vi "Actor Core.vi"(8 "error in":errorcluster, 11 "Project Builder in":refnum<class "Project Builder.lvclass">) -> (0 "error out":errorcluster, 3 "Actor out":refnum<class "Actor.lvclass">)   [LabVIEW 2014, in "Project Builder.lvclass"]
doc: "(<B>Filename</B>: Actor Framework.lvlib:Actor.lvclass:Actor Core.vi)\n\nReceives messages to the actor, reacts to them, and initiates any error handling that may shut the actor down.\n\nDescendant classes may override this VI to append parallel tasks for the actor to complete while it handles messages. Overrides use the Call Parent Method node."
uses:
  Project Builder.lvclass
  Controls/Source Code Control Selection - STYP.ctl
  Controls/Cron String - STYP.ctl
  <vilib>/ActorFramework/Actor/Actor.lvclass
  Jenkins Builder/Jenkins Builder.lvclass
  QSM/TypeDef/Invalid Option - STYP.ctl
  Project Builder.lvclass/Project Builder.ctl
  <vilib>/Utility/miscctls.llb/LVRowAndColumnTypeDef.ctl
  Shared/Controls/LabVIEW Build - STYP.ctl
  Shared/Controls/Run VI - STYP.ctl
  Actors/CI Project/CI Project.lvclass
  <vilib>/ActorFramework/Actor/Actor.lvclass/Actor.ctl
  <vilib>/ActorFramework/Message Enqueuer/Message Enqueuer.lvclass/Message Enqueuer.ctl
  Actors/Job Initialize/Job Initialize.lvclass
  Actors/CI Project/CI Project.lvclass/CI Project.ctl
  Actors/Job Initialize/Job Initialize.lvclass/Job Initialize.ctl
  Actors/Build Job/Build Job.lvclass
  Jenkins Builder Messages/Build Msg/Build Msg.lvclass/Build Msg.ctl
  Actors/CI Project/Read Build Recipe.vi
  Actors/CI Project/Read Project Name.vi
  Actors/CI Project/Read Artifact Days.vi
  Actors/CI Project/Read HostName.vi
  Actors/CI Project/Read Notification.vi
  Actors/Job Initialize/Read Build Trigger.vi
  Actors/Job Initialize/Read Source Code Poll.vi
  <vilib>/ActorFramework/Message Enqueuer/Init from Existing Queue.vi
  <vilib>/ActorFramework/Message Enqueuer/Enqueue.vi
  QSM/API/QSM - Add State(s) to Back.vi
  <vilib>/ActorFramework/Message Priority Queue/Priority Enqueue.vi
  QSM/API/QSM - Add State(s) to Front.vi
  <vilib>/ActorFramework/Message Enqueuer/Message Enqueuer.lvclass
  <vilib>/ActorFramework/Stop Msg/Stop Msg.lvclass
  Jenkins Builder Messages/Build Msg/Build Msg.lvclass
  Actors/LabVIEW Build/LabVIEW Build.lvclass
  Actors/Run VI/Run VI.lvclass
panel:
  in  "Load":bool
  in  "Save":bool
  in  "Build":bool
  in  "Main Tab":enum32{"Information", "Result Text"}(tab)
  out "Build Type Tab":enum32{"LabVIEW Build", "Run VI", "Blank"}(tab)
  in  "Title 2":string="LabVIEW Build"
  in  "Project Path":path=path "C:/Projects/LabVIEW Continuous Integration/LabVIEW Continuous Integration.lvproj"
  in  "Build Spec":u16(ring) items=["LabVIEW CI Service", "Test CI Mediator", "Test LabVIEW Launcher"]
  in  "Wait Until Done?":bool
  in  "VI Path":path=path "C:/Projects/LabVIEW Continuous Integration/LabVIEW Continuous Integration.lvproj"
  in  "Title 3":string="Run VI"
  in  "Source Code Poll":T1
  in  "Build Trigger":T2={"Day of Week"=enum."Everyday", "Hour"=23, "Enable?"=FALSE} {"Hour" min=0 max=23}
  in  "Jenkins Hostname(IP Address:Port Number)":string
  in  "Project Name":string="LabVIEW Test"
  in  "How many days to Artifact?":i32=15
  in  "Notification (Separate by Space)":string="brandyn.adderley@ni.com"
  in  "Build Steps":i32(listbox) caption="Build Steps(2)"
  in  "Add":bool
  in  "Remove":bool
  in  "Step Type":enum16{"LabVIEW Build", "Run VI"}(ring)
  out "Build Text":string
  out "Progress":u8(slide) scale=0.0..100.0
  in  "Title":string="Continuous Integration Project"
  # "<No build Steps>"
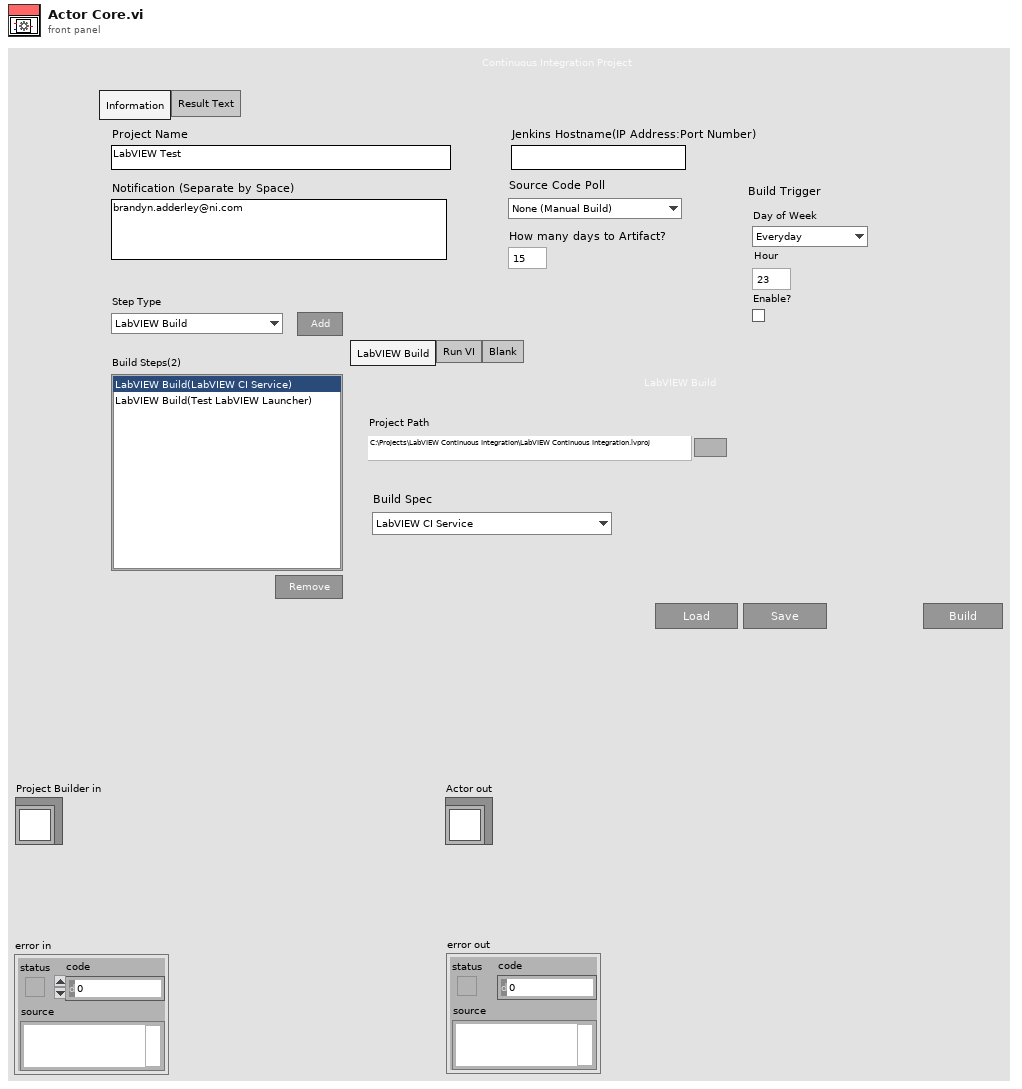
[diagram p1: front panel]
types:
  T1 = typedef "Source Code Control Selection - STYP.ctl" = enum16{"None (Manual Build)", "Every 15 Minutes", "Every 30 Minutes", "Every 45 Minutes", "Every Hour", "Every 2 Hours", "Everyday "}
  T2 = typedef "Cron String - STYP.ctl" = cluster{"Day of Week":enum16{"Everyday", "Sunday", "Monday", "Tuesday", "Wednesday", "Thursday", "Friday", "Saturday"}, "Hour":i32, "Enable?":bool}
  T3 = typedef "Invalid Option - STYP.ctl" = enum16{"Dialog", "Error", "Ignore"}
  T4 = typedef "QSM - STYP.ctl" = cluster{"Invalid Option":T3, "QSM":refnum<queue>}
  T5 = enum8{"Enabled", "Disabled", "Disabled and Grayed Out"}
  T6 = typedef "LVRowAndColumnTypeDef.ctl" = cluster{"Row":i32, "Column":i32}
  T7 = typedef "LabVIEW Build - STYP.ctl" = cluster{"Executor_Number":string, "Workspace_Path":string, "Build_Spec":string, "Project_Path":string, "Auto_Version_Increment":bool}
  T8 = typedef "Run VI - STYP.ctl" = cluster{"Executor_Number":string, "VI_Path":string, "Wait_Until_Done":bool}
  T9 = enum32{"invalid app kind", "Development System", "Run Time System", "Student Edition", "Embedded LabVIEW", "Evaluation", "Custom"}
  T10 = enum16{"open", "replace", "create", "open or create", "replace or create", "replace or create with confirmation"}
  T11 = cluster{"Core":cluster{"Current VI Reference":refnum<vi>, "Close Panel on Exit?":bool}, "Project Name":string, "Jenkins Hostname":string, "Notification":string, "How many days to Artifact?":i32, "Source Code Poll":T1, "Build Trigger":T2, "Main Tab":enum32{"Information", "Result Text"}, "Build Steps Ref":refnum<vi>, "Build Type Tab":enum32{"LabVIEW Build", "Run VI", "Blank"}, "Project Path Ref":refnum<vi>, "Build Spec":refnum<vi>, "Number of Build Steps":i32, "Step Type":enum16{"LabVIEW Build", "Run VI"}, "Active Step Data":variant, "Build Steps Data":variant, "Active GUID":string, "Build Step Index":i32, "Build Events":refnum<event-registration>, "CI Project":refnum<class "CI Project.lvclass">, "Build Text":string, "Jenkins Build Count":i32, "Jenkins Steps":i32, "Build Ref":refnum<vi>, "Load Ref":refnum<vi>, "Save Ref":refnum<vi>, "List Text":string}
  T12 = cluster{"Current VI Reference":refnum<vi>, "Close Panel on Exit?":bool}
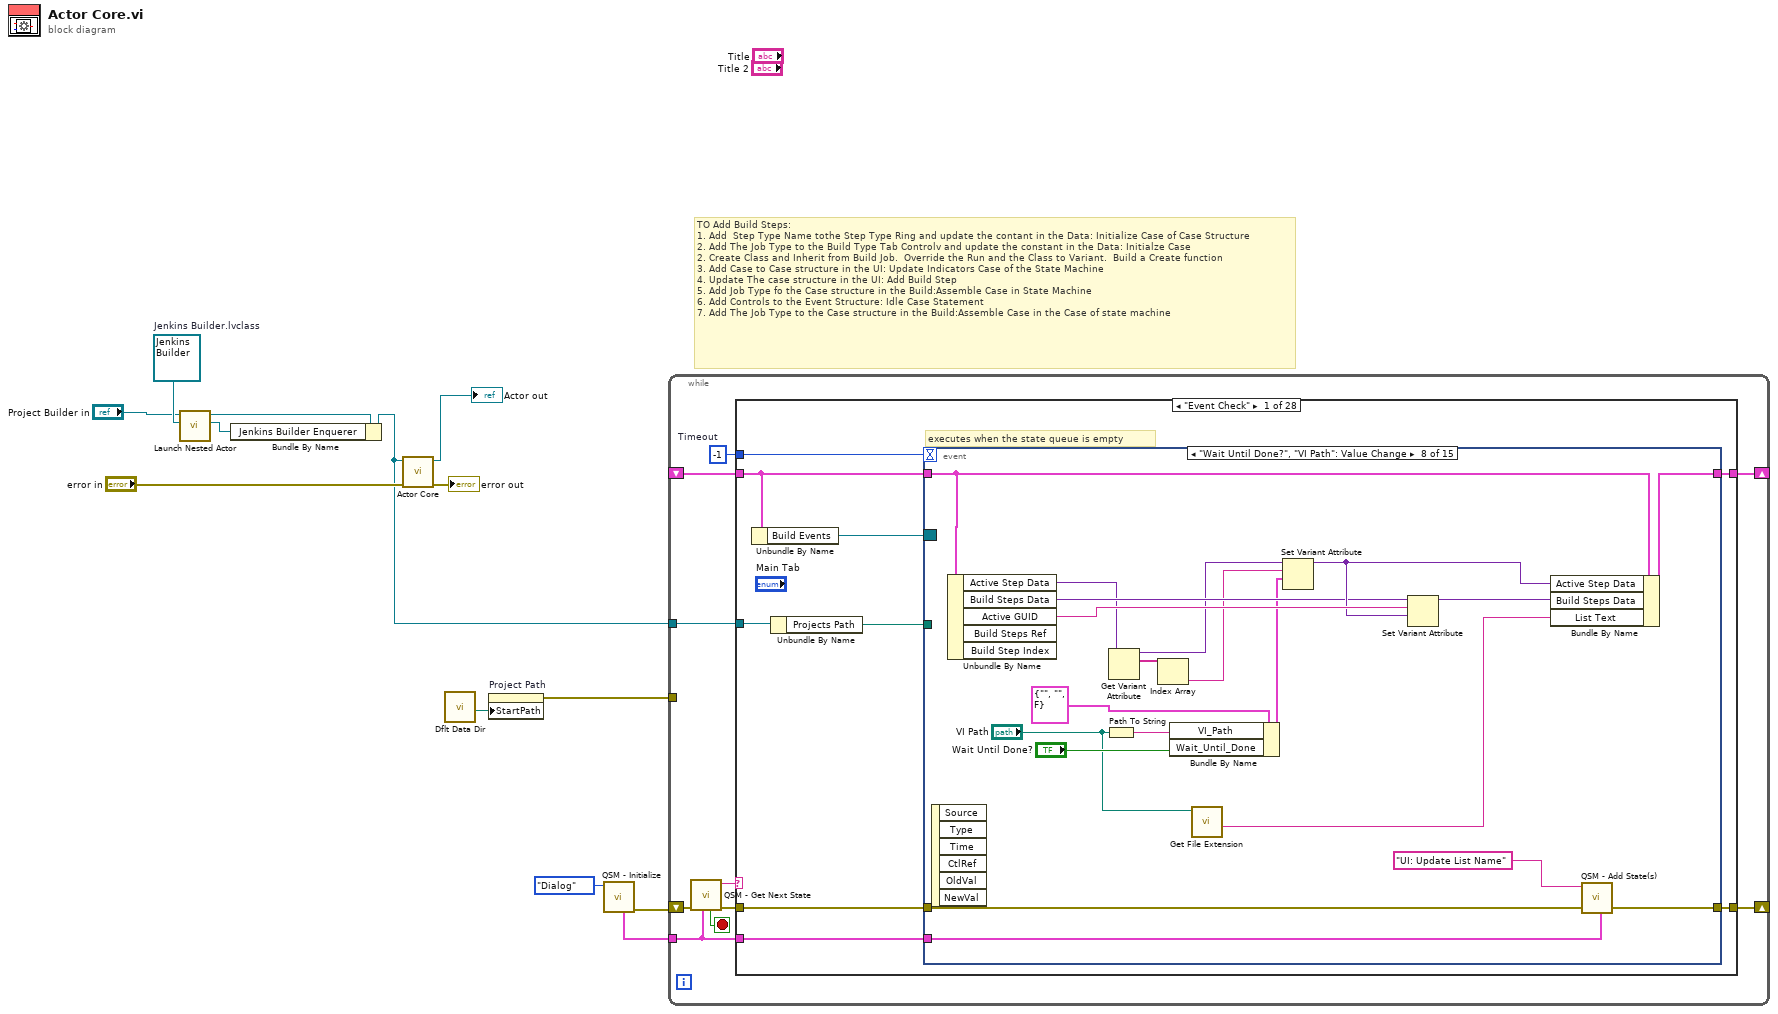
[diagram p0: block diagram]
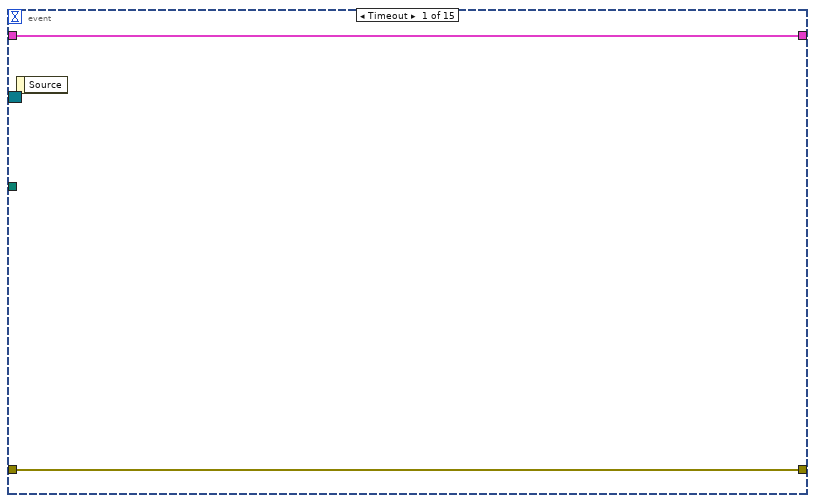
[diagram p2: hidden frame]
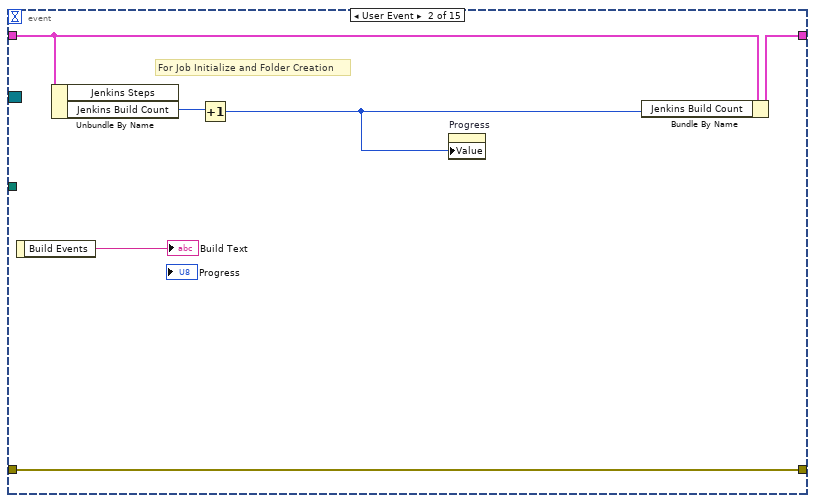
[diagram p3: hidden frame]
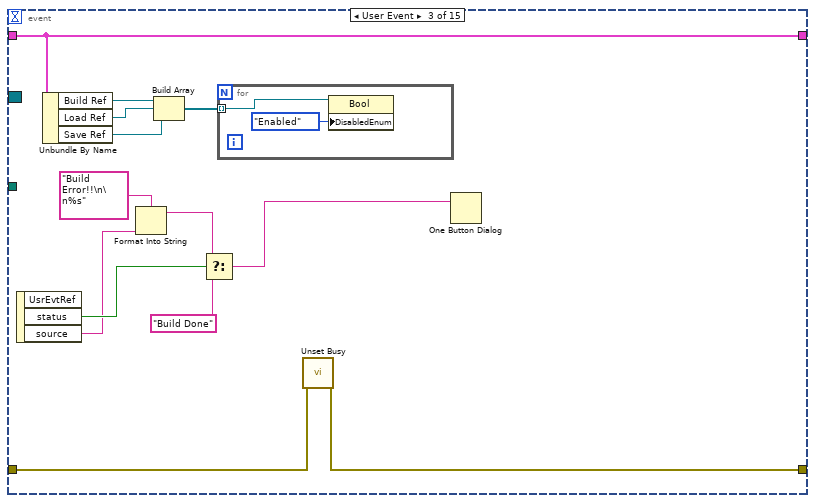
[diagram p4: hidden frame]
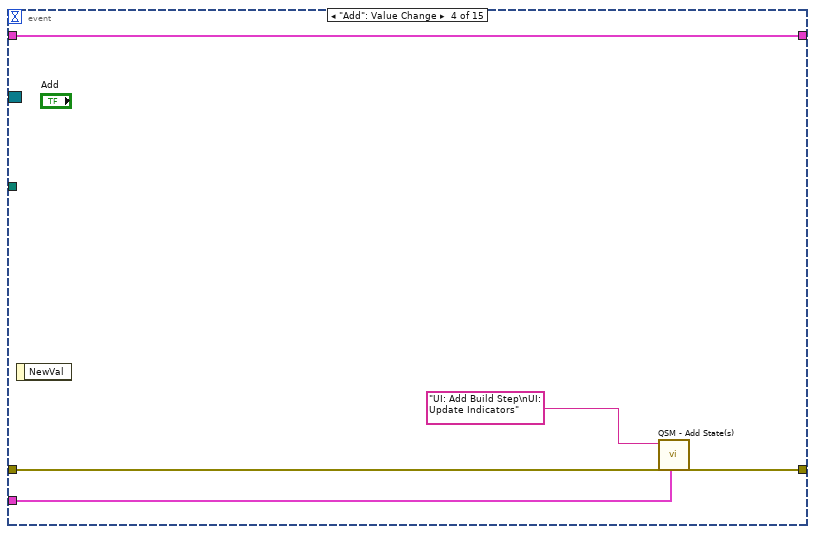
[diagram p5: hidden frame]
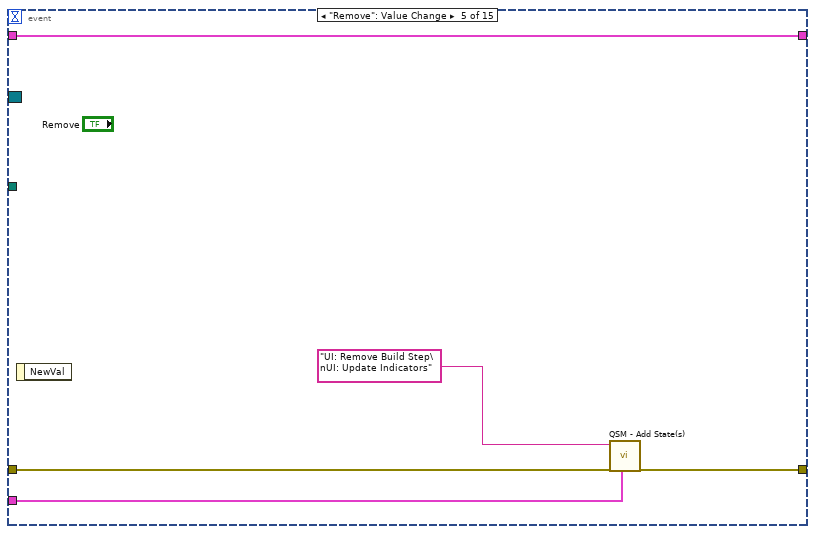
[diagram p6: hidden frame]
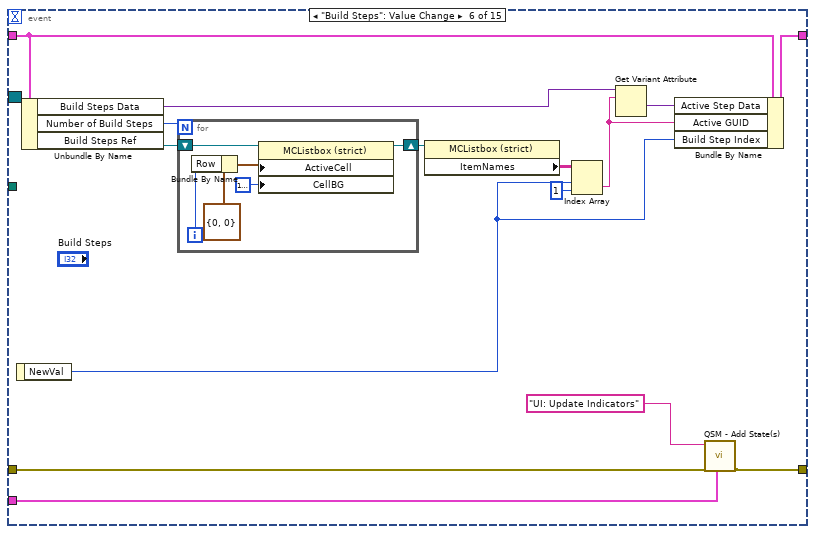
[diagram p7: hidden frame]
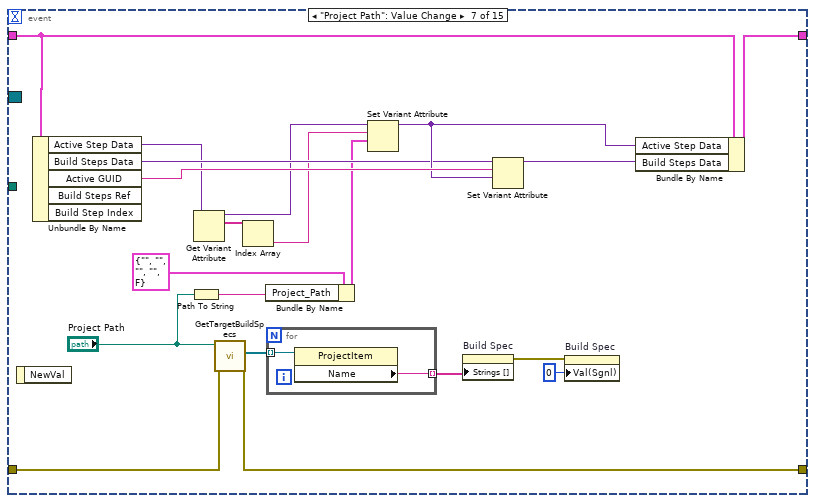
[diagram p8: hidden frame]
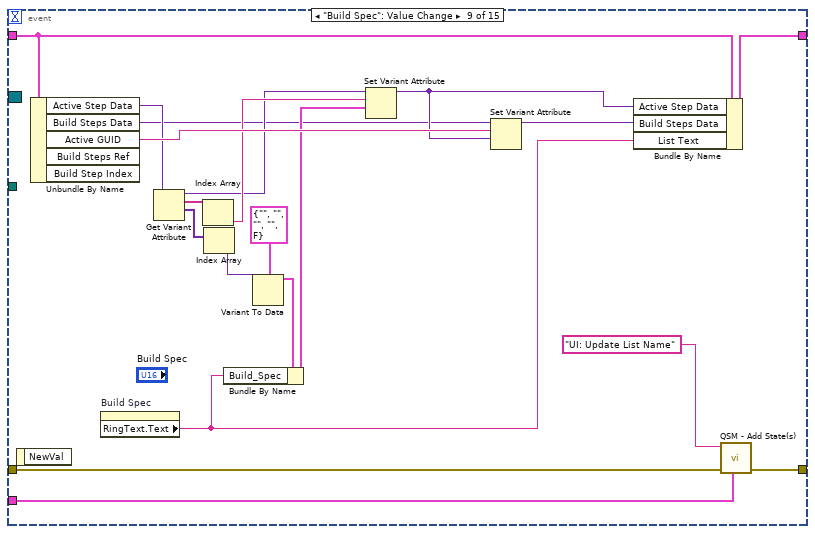
[diagram p9: hidden frame]
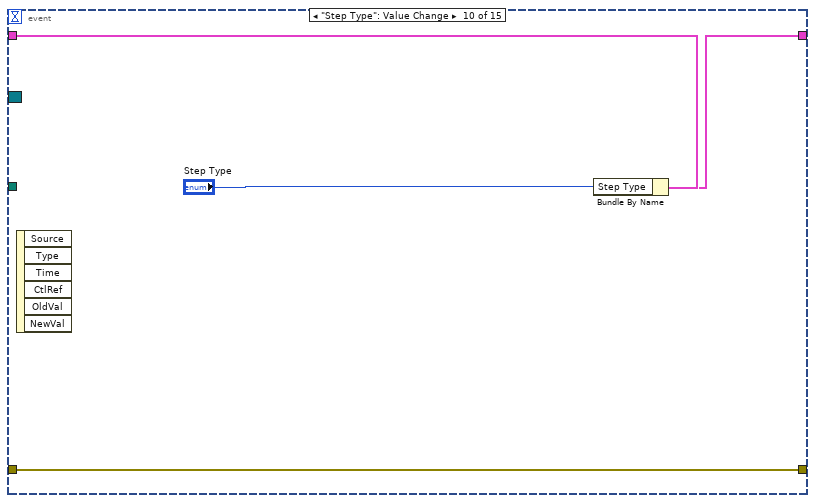
[diagram p10: hidden frame]
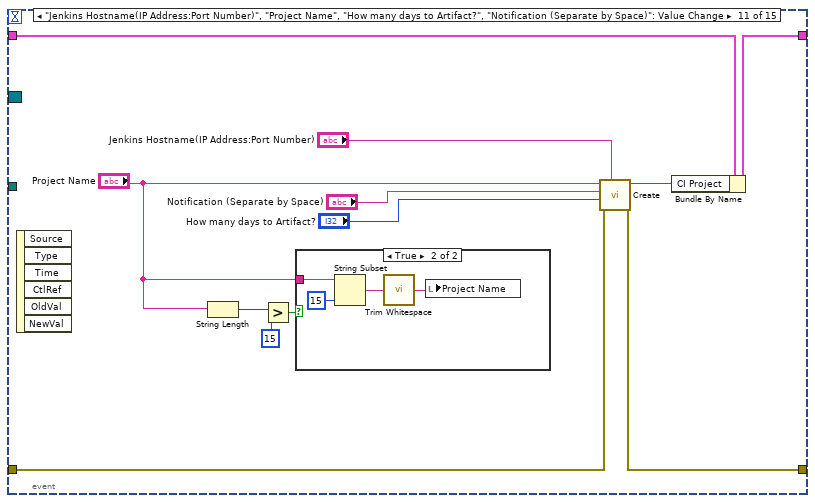
[diagram p11: hidden frame]
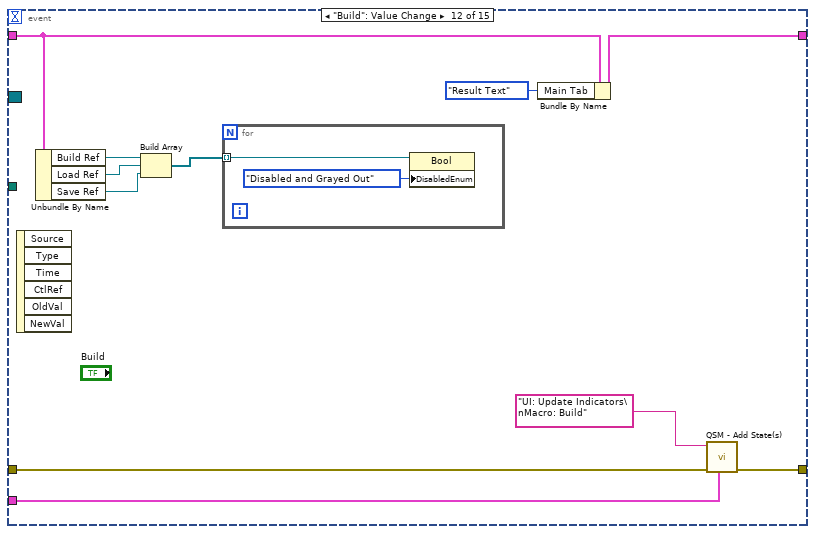
[diagram p13: hidden frame]
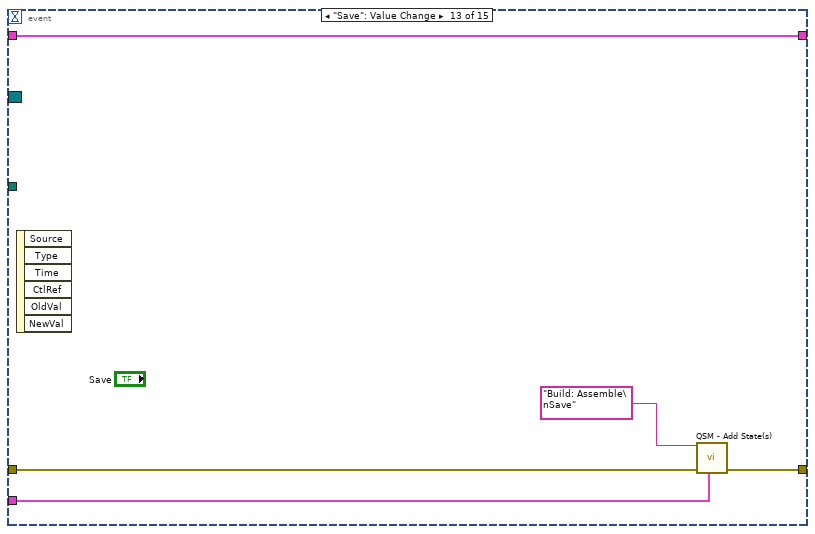
[diagram p14: hidden frame]
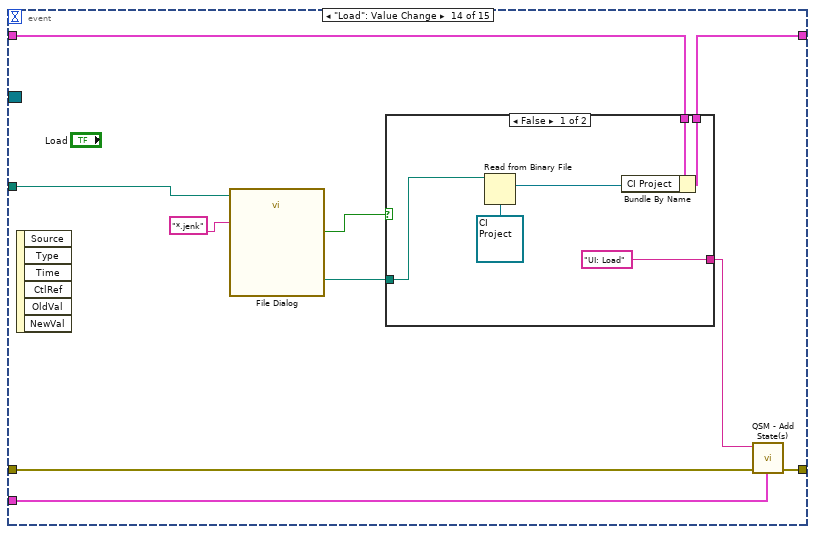
[diagram p15: hidden frame]
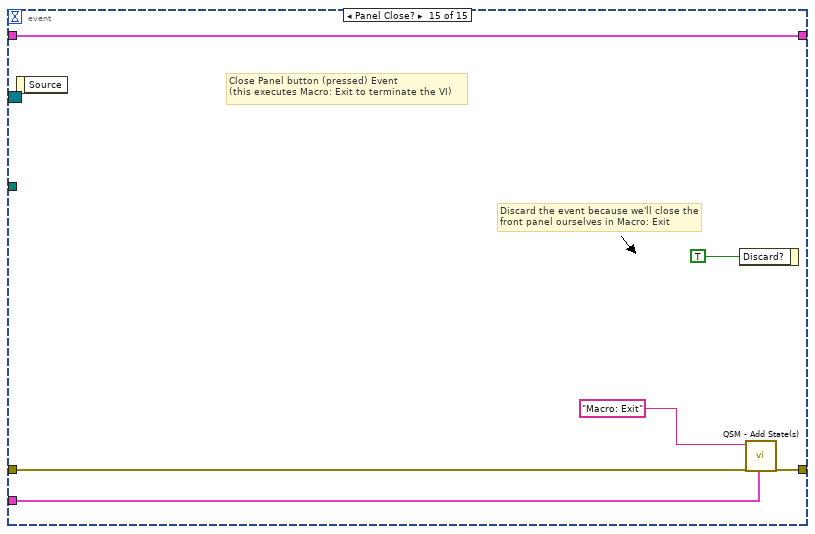
[diagram p17: hidden frame]
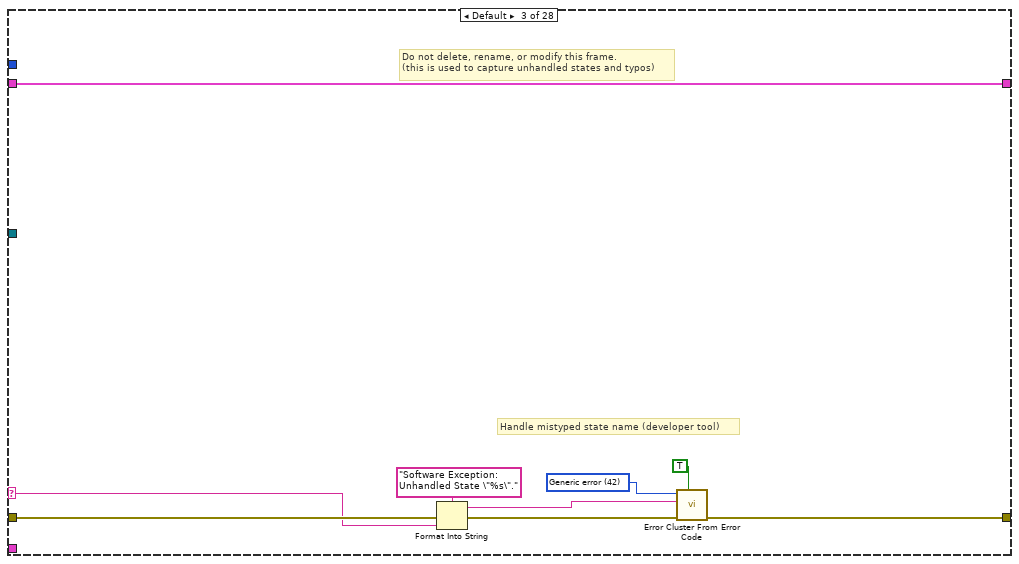
[diagram p19: hidden frame]
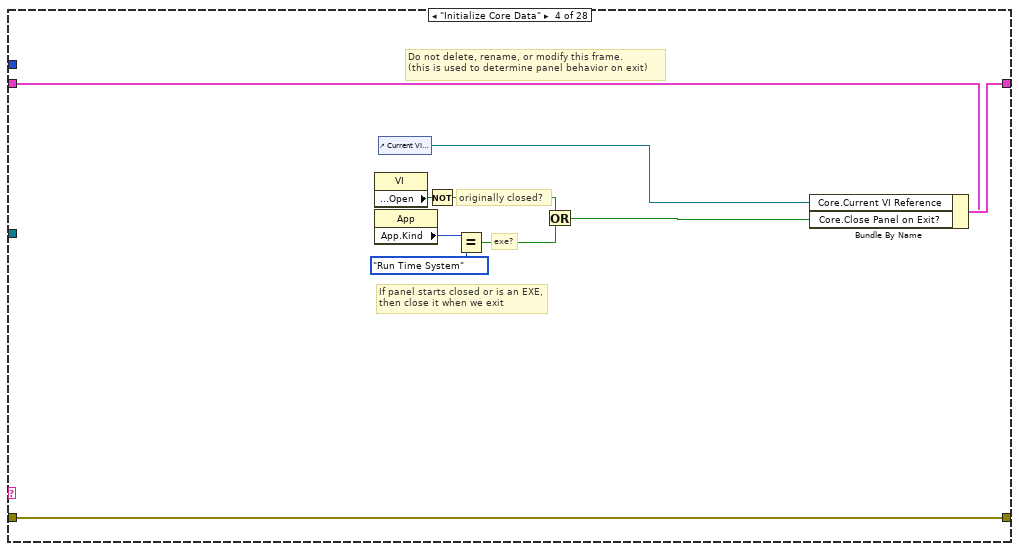
[diagram p20: hidden frame]
diagram:
  w10 = refnum<class "Jenkins Builder.lvclass"> refnum  # Jenkins Builder.lvclass
  # "TO Add Build Steps:\n1. Add  Step Type Name tothe Step Type Ring and update the contant in the Data: Initialize Case of Case Structure\n2. Add The Job Type to the Build Type Tab Controlv and update the constant in the Data: Initialze Case\n2. Create Class and Inherit from Build Job.  Override the Run and the Class to Variant.  Build a Create function\n3. Add Case to Case structure in the UI: Update Indicators Case of the State Machine\n4. Update The case structure in the UI: Add Build Step\n5. Add Job Type fo the Case structure in the Build:Assemble Case in State Machine\n6. Add Controls to the Event Structure: Idle Case Statement \n7. Add The Job Type to the Case structure in the Build:Assemble Case in the Case of state machine"
  n1 = call <vilib>:"Launch Nested Actor.vi"("Nested Actor"=w10, "Caller Actor in"="Project Builder in") -> ("Nested Actor's Enqueuer"=w6:refnum<class "Message Enqueuer.lvclass">, "Caller Actor out"=w8:refnum<class "Project Builder.lvclass">)  [unwired: 7 in, 1 out]
  n2 = Bundle By Name(cluster=w8, "Jenkins Builder Enquerer"=w6) -> (w7:refnum<class "Project Builder.lvclass">)
  n3 = call-parent "Actor Core.vi"("error in"="error in", "Actor in"=w7) -> ("error out"=→"error out":errorcluster, "Actor out"=→"Actor out":refnum<class "Actor.lvclass">)  [unwired: 8 in]
  n4 = call <vilib>:"Dflt Data Dir.vi"() -> ("App:Default Data Directory"=w2:path)
  n5 = property on="Project Path" class="Path"("StartPath"=w2) -> (error out=w1:errorcluster)  [unwired: 2 in, 1 out]
  n6 = call "QSM - Initialize.vi"("Invalid Option"=Invalid_Option_-_STYP."Dialog") -> ("Error Out"=w5:errorcluster, "QSM"=w3:T4)  [unwired: 9 in]
  n7 = while {
    shift-right: [w22] -> _
    shift-left: _ -> [w21]
    shift-right: [w23] -> _
    shift-left: w5 -> [w18]
    tunnel: w7 -> [w19]
    tunnel: w3 -> [w16]
    tunnel: w1 -> [_]
    stop <- w15 stop-if-true
    w20 = -1  # Timeout
    n8 = call "QSM - Get Next State.vi"("QSM"=w16, "error in (no error)"=w18) -> ("error out"=w17:errorcluster, "State"=w14:string, "Stop?"=w15:bool)  [unwired: 7 in]
    n9 = case shown="\"Event Check\"" w14 {
      selector: w14 -> [_ _ w212 _ _ _ _ _ _ _ _ _ _ _ _ _ _ _ _ _ _ _ _ _ _ _ _ _]
      tunnel: w21 -> [w28 w210 w214 w223 w232 w247 w248 w250 _ w281 w283 w287 w290 w314 w352 w396 w417 w445 w485 w501 w507 w512 w517 w518 w522 w537 w579 w592]
      tunnel: [w32 w211 w216 w229 errorcluster {"status"=FALSE, "code"=0, "source"=""} ("error out") w234 w249 w251 w279 w282 w284 w288 w301 w303 w365 w403 w418 w460 w487 w502 w504 w509 w514 w519 w529 w539 w576 w580] -> w23
      tunnel: w17 -> [w31 w211 w215 w229 w231 w235 w249 w251 w279 w282 w285 w288 w301 w304 w365 w403 w418 w460 w487 w502 w505 w510 w515 w519 w526 w540 w577 w582]
      tunnel: [w30 w210 w214 w230 w232 w247 w248 w250 w280 w281 w283 w287 w289 w313 w351 w395 w417 w445 w484 w501 w507 w512 w517 w518 w531 w536 w579 w592] -> w22
      tunnel: w20 -> [w29 _ _ _ _ _ _ _ _ _ _ _ _ _ _ _ _ _ _ _ _ _ _ _ _ _ _ _]
      tunnel: w19 -> [w26 _ _ _ _ w245 _ _ _ _ _ _ w300 w312 _ _ _ _ _ _ _ _ _ _ w528 _ w575 w593]
      tunnel: w16 -> [w24 _ _ _ _ w236 _ _ _ _ _ _ _ w305 _ _ _ _ _ _ w506 w511 w516 _ _ _ _ _]
      frame "Event Check" {
        # "executes when the state queue is empty"
        n10 = Unbundle By Name(w28) -> ("Build Events"=w27:refnum<event-registration>)
        n11 = Unbundle By Name(w26) -> ("Projects Path"=w25:path)
        n12 = event shown="[7] \"Wait Until Done?\", \"VI Path\": Value Change" {
          selector: w27 -> [_ _ _ _ _ _ _ _ _ _ _ _ _ _ _]
          dyn-events: _ -> [_ _ _ _ _ _ _ _ _ _ _ _ _ _ _]
          timeout: w29 -> [_ _ _ _ _ _ _ _ _ _ _ _ _ _ _]
          tunnel: w28 -> [w33 w37 w51 w60 w65 w75 w95 w120 w148 w151 w158 w177 w186 w195 w209]
          tunnel: [w34 w40 w52 w57 w63 w67 w104 w110 w130 w152 w160 w170 w183 w188 w205] -> w32
          tunnel: w31 -> [w34 w40 w53 w58 w64 w68 w105 w111 w131 w152 w161 w171 w184 w189 w206]
          tunnel: [w33 w36 w51 w60 w65 w74 w94 w119 w147 w150 w157 w178 w186 w194 w209] -> w30
          tunnel: w25 -> [_ _ _ _ _ _ _ _ _ _ _ _ _ w192 _]
          tunnel: w24 -> [_ _ _ w59 w62 w69 _ w112 w132 _ _ w172 w185 w190 w207]
          event Timeout {
            n13 = event-data() -> ()  [unwired: 1 in, 1 out]
          }
          event User Event {
            # "For Job Initialize and Folder Creation"
            n14 = event-data() -> ("Build Events"=→"Build Text":string)  [unwired: 1 in]
            n15 = Unbundle By Name(w37) -> ("Jenkins Build Count"=w38:i32)  [unwired: 1 out]
            n16 = Increment(x=w38) -> (x+1=w35:i32)
            n17 = property on="Progress" class="Slide (strict)"("Value"=w35) -> ()  [unwired: 2 in, 2 out]
            n18 = Bundle By Name(cluster=w37, "Jenkins Build Count"=w35) -> (w36:T11)
          }
          event User Event {
            n19 = event-data() -> ("status"=w46:bool, "source"=w43:string)  [unwired: 1 in, 1 out]
            n20 = Unbundle By Name(w51) -> ("Build Ref"=w50:refnum<vi>, "Load Ref"=w49:refnum<vi>, "Save Ref"=w48:refnum<vi>)
            n21 = Format Into String(format string="Build Error!!\n\n%s", w43) -> (resulting string=w42:string)  [unwired: 2 in, 1 out]
            n22 = Build Array(w50, w49, w48) -> (w47:refnum<vi>[])
            n23 = Select(t=w42, s=w46, f="Build Done" ("message")) -> (s? t:f=w41:string)
            n24 = for {
              tunnel: w47 -> [w54] mode=indexing
              n25 = property class="Bool"(reference=w54, "DisabledEnum"=T5."Enabled" ("Disabled")) -> ()  [unwired: 1 in, 2 out]
            }
            n26 = call <vilib>:"Unset Busy.vi"("error in (no error)"=w53) -> ("error out"=w52:errorcluster)  [unwired: 10 in]
            n27 = One Button Dialog(message=w41) -> ()  [unwired: 1 in, 1 out]
          }
          event "Add": Value Change {
            n28 = event-data() -> ()  [unwired: 1 in, 1 out]
            n29 = call-poly "QSM - Add State(s).vi"("QSM"=w59, "error in (no error)"=w58, "State(s)"="UI: Add Build Step\nUI: Update Indicators" ("State(s) at Back (\"\")")) -> ("error out"=w57:errorcluster)  [unwired: 8 in]
          }
          event "Remove": Value Change {
            n30 = event-data() -> ()  [unwired: 1 in, 1 out]
            n31 = call-poly "QSM - Add State(s).vi"("QSM"=w62, "error in (no error)"=w64, "State(s)"="UI: Remove Build Step\nUI: Update Indicators" ("State(s) at Back (\"\")")) -> ("error out"=w63:errorcluster)  [unwired: 8 in]
          }
          event "Build Steps": Value Change {
            n32 = event-data() -> ("NewVal"=w70:i32)  [unwired: 1 in]
            n33 = Unbundle By Name(w75) -> ("Build Steps Data"=w73:variant, "Number of Build Steps"=w79:i32, "Build Steps Ref"=w80:refnum<vi>)
            n34 = for {
              N: w79 -> [_]
              shift-right: [w84] -> w78
              shift-left: w80 -> [w85]
              i -> [w81]
              n35 = Bundle By Name(cluster=T6 {"Row"=0, "Column"=0} ("Active Cell:Active Cell"), "Row"=w81) -> (w82:T6)
              n36 = property class="MCListbox (strict)"(reference=w85, "ActiveCell"=w82, "CellBG"=u32 16777225) -> (reference out=w84:refnum<vi>)  [unwired: 1 in, 1 out]
            }
            n37 = property class="MCListbox (strict)"(reference=w78) -> ("ItemNames"=w77:string[][])  [unwired: 1 in, 2 out]
            n38 = Index Array(array=w77, index (row)=w70, index (col)=1 ("disabled index (col)")) -> (element=w71:string)
            n39 = Get Variant Attribute(Variant=w73, name=w71) -> (value=w72:variant)  [unwired: 2 in, 3 out]
            n40 = Bundle By Name(cluster=w75, "Active Step Data"=w72, "Active GUID"=w71, "Build Step Index"=w70) -> (w74:T11)
            n41 = call-poly "QSM - Add State(s).vi"("QSM"=w69, "error in (no error)"=w68, "State(s)"="UI: Update Indicators" ("State(s) at Back (\"\")")) -> ("error out"=w67:errorcluster)  [unwired: 8 in]
          }
          event "Project Path": Value Change {
            n42 = event-data() -> ()  [unwired: 1 in, 1 out]
            n43 = Unbundle By Name(w95) -> ("Active Step Data"=w99:variant, "Build Steps Data"=w100:variant, "Active GUID"=w103:string)  [unwired: 2 out]
            n44 = Path To String(path="Project Path") -> (string=w90:string)
            n45 = Get Variant Attribute(Variant=w99) -> (duplicate Variant=w97:variant, names=w98:string[])  [unwired: 3 in, 2 out]
            n46 = call <vilib>:"GetTargetBuildSpecs.vi"("error in (no error)"=w105, "Path to project"="Project Path") -> ("error out"=w104:errorcluster, "buildspec refs"=w106:refnum<vi>[])  [unwired: 7 in, 1 out]
            n47 = Index Array(array=w98) -> (element=w96:string)  [unwired: 1 in]
            n48 = Bundle By Name(cluster=T7 {"Executor_Number"="", "Workspace_Path"="", "Build_Spec"="", "Project_Path"="", "Auto_Version_Increment"=FALSE} ("LabVIEW Build"), "Project_Path"=w90) -> (w92:T7)
            n49 = for {
              tunnel: w106 -> [w108] mode=indexing
              tunnel: [w107] -> w89 mode=indexing
              n50 = property class="ProjectItem"(reference=w108) -> ("Name"=w107:string)  [unwired: 1 in, 2 out]
            }
            n51 = Set Variant Attribute(Variant=w97, name=w96, value=w92) -> (Variant out=w101:variant)  [unwired: 1 in, 2 out]
            n52 = property on="Build Spec" class="Ring (strict)"("Strings []"=w89) -> (error out=w87:errorcluster)  [unwired: 2 in, 1 out]
            n53 = Set Variant Attribute(Variant=w100, name=w103, value=w101) -> (Variant out=w102:variant)  [unwired: 1 in, 2 out]
            n54 = property on="Build Spec" class="Ring (strict)"(error in=w87, "Val(Sgnl)"=u16 0 ("Value (Signaling)")) -> ()  [unwired: 1 in, 2 out]
            n55 = Bundle By Name(cluster=w95, "Active Step Data"=w101, "Build Steps Data"=w102) -> (w94:T11)
          }
          event "Wait Until Done?", "VI Path": Value Change {
            n56 = event-data() -> ()  [unwired: 1 in, 6 out]
            n57 = Unbundle By Name(w120) -> ("Active Step Data"=w124:variant, "Build Steps Data"=w125:variant, "Active GUID"=w128:string)  [unwired: 2 out]
            n58 = Path To String(path="VI Path") -> (string=w117:string)
            n59 = Get Variant Attribute(Variant=w124) -> (duplicate Variant=w122:variant, names=w123:string[])  [unwired: 3 in, 2 out]
            n60 = Index Array(array=w123) -> (element=w121:string)  [unwired: 1 in]
            n61 = Bundle By Name(cluster=T8 {"Executor_Number"="", "VI_Path"="", "Wait_Until_Done"=FALSE} ("Run VI"), "VI_Path"=w117, "Wait_Until_Done"="Wait Until Done?") -> (w118:T8)
            n62 = call <vilib>:"Get File Extension.vi"("file"="VI Path") -> ("filename without extension"=w113:string)  [unwired: 7 in, 3 out]
            n63 = Set Variant Attribute(Variant=w122, name=w121, value=w118) -> (Variant out=w126:variant)  [unwired: 1 in, 2 out]
            n64 = Set Variant Attribute(Variant=w125, name=w128, value=w126) -> (Variant out=w127:variant)  [unwired: 1 in, 2 out]
            n65 = Bundle By Name(cluster=w120, "Active Step Data"=w126, "Build Steps Data"=w127, "List Text"=w113) -> (w119:T11)
            n66 = call-poly "QSM - Add State(s).vi"("QSM"=w112, "error in (no error)"=w111, "State(s)"="UI: Update List Name") -> ("error out"=w110:errorcluster)  [unwired: 8 in]
          }
          event "Build Spec": Value Change {
            n67 = event-data() -> ()  [unwired: 1 in, 1 out]
            n68 = Unbundle By Name(w148) -> ("Active Step Data"=w144:variant, "Build Steps Data"=w138:variant, "Active GUID"=w146:string)  [unwired: 2 out]
            n69 = property on="Build Spec" class="Ring (strict)"() -> ("RingText.Text"=w133:string)  [unwired: 2 in, 2 out]
            n70 = Get Variant Attribute(Variant=w144) -> (duplicate Variant=w139:variant, names=w143:string[], values=w137:variant[])  [unwired: 3 in, 1 out]
            n71 = Index Array(array=w143) -> (element=w142:string)  [unwired: 1 in]
            n72 = Index Array(array=w137) -> (element=w136:variant)  [unwired: 1 in]
            n73 = Variant To Data(type=T7 {"Executor_Number"="", "Workspace_Path"="", "Build_Spec"="", "Project_Path"="", "Auto_Version_Increment"=FALSE} ("LabVIEW Build"), Variant=w136) -> (data=w134:T7)  [unwired: 1 in, 1 out]
            n74 = Bundle By Name(cluster=w134, "Build_Spec"=w133) -> (w141:T7)
            n75 = Set Variant Attribute(Variant=w139, name=w142, value=w141) -> (Variant out=w140:variant)  [unwired: 1 in, 2 out]
            n76 = Set Variant Attribute(Variant=w138, name=w146, value=w140) -> (Variant out=w145:variant)  [unwired: 1 in, 2 out]
            n77 = Bundle By Name(cluster=w148, "Active Step Data"=w140, "Build Steps Data"=w145, "List Text"=w133) -> (w147:T11)
            n78 = call-poly "QSM - Add State(s).vi"("QSM"=w132, "error in (no error)"=w131, "State(s)"="UI: Update List Name" ("State(s) at Back (\"\")")) -> ("error out"=w130:errorcluster)  [unwired: 8 in]
          }
          event "Step Type": Value Change {
            n79 = event-data() -> ()  [unwired: 1 in, 6 out]
            n80 = Bundle By Name(cluster=w151, "Step Type"="Step Type") -> (w150:T11)
          }
          event "Jenkins Hostname(IP Address:Port Number)", "Project Name", "How many days to Artifact?", "Notification (Separate by Space)": Value Change {
            n81 = event-data() -> ()  [unwired: 1 in, 6 out]
            n82 = String Length(string="Project Name") -> (length=w156:i32)
            n83 = Greater?(x=w156, y=15) -> (0:w154:bool)
            n84 = case shown="True" w154 {
              tunnel: "Project Name" -> [_ w168]
              frame False {
              }
              frame True {
                n85 = String Subset(string=w168, length (rest)=15 ("length (rest)")) -> (substring=w166:string)  [unwired: 1 in]
                n86 = call <vilib>:"Trim Whitespace.vi"("string"=w166) -> ("trimmed string"=w165:string)  [unwired: 1 in]
                n87 = local write "Project Name"(w165) -> ()
              }
            }
            n88 = call "Create.vi"("HostName"="Jenkins Hostname(IP Address:Port Number)", "error in (no error)"=w161, "Artifact Days"="How many days to Artifact?", "Notification"="Notification (Separate by Space)", "Project Name"="Project Name") -> ("error out"=w160:errorcluster, "CI Project out"=w159:refnum<class "CI Project.lvclass">)  [unwired: 5 in]
            n89 = Bundle By Name(cluster=w158, "CI Project"=w159) -> (w157:T11)
          }
          event "Build": Value Change {
            n90 = event-data() -> ()  [unwired: 1 in, 6 out]
            n91 = Unbundle By Name(w177) -> ("Build Ref"=w174:refnum<vi>, "Load Ref"=w176:refnum<vi>, "Save Ref"=w175:refnum<vi>)
            n92 = Build Array(w174, w176, w175) -> (w173:refnum<vi>[])
            n93 = for {
              tunnel: w173 -> [w180] mode=indexing
              n94 = property class="Bool"(reference=w180, "DisabledEnum"=T5."Disabled and Grayed Out" ("Disabled")) -> ()  [unwired: 1 in, 2 out]
            }
            n95 = Bundle By Name(cluster=w177, "Main Tab"=enum32{"Information", "Result Text"}."Result Text") -> (w178:T11)
            n96 = call-poly "QSM - Add State(s).vi"("QSM"=w172, "error in (no error)"=w171, "State(s)"="UI: Update Indicators\nMacro: Build") -> ("error out"=w170:errorcluster)  [unwired: 8 in]
          }
          event "Save": Value Change {
            n97 = event-data() -> ()  [unwired: 1 in, 6 out]
            n98 = call-poly "QSM - Add State(s).vi"("QSM"=w185, "error in (no error)"=w184, "State(s)"="Build: Assemble\nSave") -> ("error out"=w183:errorcluster)  [unwired: 8 in]
          }
          event "Load": Value Change {
            n99 = event-data() -> ()  [unwired: 1 in, 6 out]
            n100 = call "File Dialog"("start path"=w192, "pattern (all files)"="*.jenk" ("pattern label")) -> ("selected path"=w196:path, "cancelled"=w193:bool)  [unwired: 10 in, 2 out]
            n101 = case shown="False" w193 {
              tunnel: w196 -> [w201 _]
              tunnel: w195 -> [w200 w203]
              tunnel: [w198 w203] -> w194
              tunnel: ["UI: Load" _] -> w187
              frame False {
                n102 = Read from Binary File(5:refnum<class "CI Project.lvclass"> refnum ("CI Project out"), 11:w201) -> (2:w199:refnum<class "CI Project.lvclass">)  [unwired: 4 in, 3 out]
                n103 = Bundle By Name(cluster=w200, "CI Project"=w199) -> (w198:T11)
              }
              frame True {
              }
            }
            n104 = call-poly "QSM - Add State(s).vi"("QSM"=w190, "error in (no error)"=w189, "State(s)"=w187) -> ("error out"=w188:errorcluster)  [unwired: 8 in]
          }
          event Panel Close? {
            # "Discard the event because we'll close the front panel ourselves in Macro: Exit"
            # "Close Panel button (pressed) Event\n(this executes Macro: Exit to terminate the VI)"
            n105 = event-data() -> ()  [unwired: 1 in, 1 out]
            n106 = event-data("Discard?"=TRUE) -> ()  [unwired: 1 in, 1 out]
            n107 = call-poly "QSM - Add State(s).vi"("QSM"=w207, "error in (no error)"=w206, "State(s)"="Macro: Exit") -> ("error out"=w205:errorcluster)  [unwired: 8 in]
          }
        }
      }
      frame "---------- Core ----------" {
        # "Do not put any code in this frame.\n(it is a separator no-op)"
      }
      frame Default {
        w219 = 42 items=["No error", "Argument error", "Memory is full", "Out of zone", "End of file", "File already open", "Generic file I/O error", "File not found", "File permission error", "Disk is full", "Duplicate path", "Too many files open", "System feature not enabled", "Resource file not found", "Cannot add resource", "Resource not found", "Image not found", "Image memory error", "Pen does not exist", "Config type invalid", "Config token not found", "Config parse error", "Config memory error", "Bad external code format", "Bad external code offset", "External code not present", "Null window", "Destroy window error", "Null menu", "Print aborted", "Bad print record", "Print driver error", "Windows error during printing", "Memory error during printing", "Print dialog error", "Generic print error", "Invalid device refnum", "Device not found", "Device parameter error", "Device unit error", "Cannot open device", "Device call aborted", "Generic error", "Cancelled by user", "Object ID too low", "Object ID too high", "Object not in heap", "Unknown heap", "Unknown object (invalid DefProc)", "Unknown object (DefProc not in table)", "Message out of range", "Invalid (null) method", "Unknown message", "Manager call not supported", "Bad address", "Network operation in progress", "Network operation timed out", "Connection is busy", "Network attribute not supported", "Network error", "Address in use", "System out of memory", "Connection aborted", "Connection refused", "Not connected", "Already connected", "Connection closed", "Initialization error (interapplication manager)", "Bad occurrence", "Wait on unbound occurrence handler", "Occurrence queue overflow", "Datalog type conflict", "Unused", "Unrecognized type (interapplication manager)", "Memory corrupt", "Failed to make temporary DLL", "Old CIN version", "Drag socket not found", "Failed to load drop-object", "Failed to register OLE object", "Failed to release OLE object", "Format specifier type mismatch", "Unknown format specifier", "Too few format specifiers", "Too many format specifiers", "Scan failed", "Newer CIN version", "Error converting to variant", "Runtime menu error", "Password tampered", "Variant attribute not found", "Incompatible variant data type", "Event data is not available", "Event Store is not present", "Occurrence is not found", "Event Queue is not created", "Event info is not available", "Refnum passed is NULL", "Error retrieving Class GUID", "Error retrieving CoClass GUID", "Error retrieving TypeLib GUID.", "Bad built application magic bytes.", "Specific driver is different from the specific driver associated with the Logical Name.", "There is no session opened to the class driver.", "Max Error", "MAX - Error with config objects", "MAX - Error loading configuration", "MAX - Group not supported"]
        # "Do not delete, rename, or modify this frame.\n(this is used to capture unhandled states and typos)"
        # "Handle mistyped state name (developer tool)"
        n108 = Format Into String(format string="Software Exception: Unhandled State \"%s\"." ("message"), error in=w215, w212) -> (resulting string=w218:string, error out=w217:errorcluster)  [unwired: 1 in]
        n109 = call <vilib>:"Error Cluster From Error Code.vi"("show call chain? (False)"=TRUE, "error in (no error)"=w217, "error message (\"\")"=w218, "error code (0)"=w219) -> ("error out"=w216:errorcluster)  [unwired: 5 in]
      }
      frame "Initialize Core Data" {
        # "Do not delete, rename, or modify this frame.\n(this is used to determine panel behavior on exit)"
        # "originally closed?"
        # "exe?"
        # "If panel starts closed or is an EXE, then close it when we exit"
        n110 = property class="VI"() -> ("Front Panel.Open"=w228:bool)  [unwired: 2 in, 2 out]
        n111 = property class="App"() -> ("App.Kind"=w227:T9)  [unwired: 2 in, 2 out]
        n112 = control-ref of="Current VI Reference"() -> (w221:refnum<vi>)
        n113 = Not(x=w228) -> (.not. x?=w225:bool)
        n114 = Equal?(x=w227, y=T9."Run Time System" ("Application:Kind")) -> (x = y?=w224:bool)
        n115 = Or(x=w225, y=w224) -> (x .or. y?=w222:bool)
        n116 = Bundle By Name(cluster=w223, "Core.Current VI Reference"=w221, "Core.Close Panel on Exit?"=w222) -> (w230:T11)
      }
      frame "Error Handler" {
        # "Unhandled Error -- Display it"
        # "Handle any errors here.\nYou can also output any states to clean-up after errors occur"
        # "Clear error"
        n117 = call <vilib>:"General Error Handler.vi"("error in (no error)"=w231) -> ()  [unwired: 10 in, 5 out]
      }
      frame "Exit" {
        (unwired) TRUE
        # "Do not put any code in this frame.\n(No errors that occur here will be handled.)"
        n118 = Unbundle By Name(w245) -> ("Main Info Path"=w240:refnum<file>)
        n119 = local read "Jenkins Hostname(IP Address:Port Number)"() -> (w244:string)
        n120 = local read "Notification (Separate by Space)"() -> (w243:string)
        n121 = call "QSM - Stop.vi"("QSM"=w236, "error in (no error)"=w235) -> ("error out"=w234:errorcluster)  [unwired: 1 in, 8 out]
        n122 = call <vilib>:"Read Self Enqueuer.vi"("Actor"=w245) -> ("Self Enqueuer"=w246:refnum<class "Message Enqueuer.lvclass">)  [unwired: 10 in]
        n123 = call <vilib>:"Send Normal Stop.vi"("Message Enqueuer"=w246) -> ()  [unwired: 10 in, 1 out]
        n124 = Build Array(w244, w243) -> (w242:string[])
        n125 = Array To Spreadsheet String(array=w242, 3:"" ("format string")) -> (spreadsheet string=w239:string)  [unwired: 1 in]
        n126 = Write to Text File(file (use dialog)=w240, text=w239) -> (refnum out=w238:refnum<file>, error out=w237:errorcluster)  [unwired: 2 in, 1 out]
        n127 = Close File(refnum=w238, error in=w237) -> ()  [unwired: 2 out]
      }
      frame "VI STOP" {
      }
      frame "---------- Data ----------" {
        # "Do not put any code in this frame.\n(It is a separator no-op. You can make a copy of this frame to create a new Data frame)"
      }
      frame "Data: Initialize" {
        w252 = refnum<event-registration> refnum  # Build Events
        w253 = ""  # List Text
        w254 = enum32{"LabVIEW Build", "Run VI", "Blank"}."Run VI"  # Build Type Tab
        w255 = enum16{"LabVIEW Build", "Run VI"}."LabVIEW Build"  # Step Type
        w259 = 0  # Jenkins Steps
        w260 = 0  # Jenkins Build Count
        w261 = ""  # Build Text
        w262 = refnum<class "CI Project.lvclass"> refnum  # CI Project
        w263 = 0  # Build Step Index
        w264 = ""  # Active GUID
        w266 = variant  # Build Steps Data
        w267 = variant  # Active Step Data
        w268 = 0  # Number of Build Steps
        w271 = T2 {"Day of Week"=enum."Everyday", "Hour"=23, "Enable?"=TRUE}  # Build Trigger
        w272 = Source_Code_Control_Selection_-_STYP."None (Manual Build)"  # Source Code Poll
        w273 = 0  # How many days to Artifact?
        w274 = ""  # Notification
        w275 = ""  # Jenkins Hostname
        w276 = ""  # Project Name
        w277 = enum32{"Information", "Result Text"}."Information"  # Main Tab
        w278 = T12 {"Current VI Reference"=refnum, "Close Panel on Exit?"=FALSE}  # Core
        # "Initialize the shift-register data, here.\n(data names are defined by what you wire into the bundle function)"
        n128 = control-ref of="Build Steps Ref"() -> (w270:refnum<vi>)
        n129 = control-ref of="Project Path Ref"() -> (w265:refnum<vi>)
        n130 = control-ref of="Build Spec"() -> (w269:refnum<vi>)
        n131 = control-ref of="Save Ref"() -> (w256:refnum<vi>)
        n132 = control-ref of="Load Ref"() -> (w257:refnum<vi>)
        n133 = control-ref of="Build Ref"() -> (w258:refnum<vi>)
        n134 = Bundle("Core"=w278, "Project Name"=w276, "Jenkins Hostname"=w275, "Notification"=w274, "How many days to Artifact?"=w273, "Source Code Poll"=w272, "Build Trigger"=w271, "Main Tab"=w277, "Build Steps Ref"=w270, "Build Type Tab"=w254, "Project Path Ref"=w265, "Build Spec"=w269, "Number of Build Steps"=w268, "Step Type"=w255, "Active Step Data"=w267, "Build Steps Data"=w266, "Active GUID"=w264, "Build Step Index"=w263, "Build Events"=w252, "CI Project"=w262, "Build Text"=w261, "Jenkins Build Count"=w260, "Jenkins Steps"=w259, "Build Ref"=w258, "Load Ref"=w257, "Save Ref"=w256, "List Text"=w253) -> (w280:T11)  [unwired: 1 in]
      }
      frame "Data: Project Select" {
      }
      frame "Data: Cleanup" {
        # "Cleanup any data and references, here.\n(this is called automatically, by the Macro: Exit)"
        n135 = Unbundle By Name(w283) -> ("Core.Current VI Reference"=w286:refnum<vi>)
        n136 = Close Reference(reference=w286, error in (no error)=w285) -> (error out=w284:errorcluster)
      }
      frame "---------- UI ----------" {
        # "Do not put any code in this frame.\n(It is a separator no-op. You can make a copy of this frame to create a new UI frame)"
      }
      frame "UI: Main Info" {
        w294 = 0 ("disabled index (row)")
        n137 = Unbundle By Name(w300) -> ("Main Info Path"=w299:refnum<file>)
        n138 = Read from Text File(file (use dialog)=w299) -> (text=w298:string)  [unwired: 3 in, 3 out]
        n139 = Spreadsheet String To Array(format string="", spreadsheet string=w298, array type (2D Dbl)="") -> (array=w296:string[][])  [unwired: 1 in]
        n140 = Index Array(array=w296, index (row)=w294, index (col)=w294) -> (element=w292:string)
        n141 = Index Array(array=w296, index (row)=w294, index (col)=1 ("disabled index (col)")) -> (element=w291:string)
        n142 = local write "Notification (Separate by Space)"(w291) -> ()
        n143 = local write "Jenkins Hostname(IP Address:Port Number)"(w292) -> ()
        n144 = Bundle By Name(cluster=w290, "Jenkins Hostname"=w292, "Notification"=w291) -> (w289:T11)
      }
      frame "UI: Initialize" {
        # "Initialize the User Interface, here.\n(this is called automatically, by the Macro: Init)"
        n145 = Unbundle By Name(w314) -> ("Core.Current VI Reference"=w306:refnum<vi>, "Build Ref"=w321:refnum<vi>, "Build Steps Ref"=w325:refnum<vi>)
        n146 = Unbundle By Name(w312) -> ("Projects Path"=w311:path)
        n147 = property class="App"() -> ("Project"=w319:refnum<vi>[])  [unwired: 2 in, 2 out]
        n148 = Index Array(array=w319) -> (element=w318:refnum<vi>)  [unwired: 1 in]
        n149 = call <vilib>:"Recursive File List.vi"("Folder Path"=w311) -> ("All Files in Dir"=w307:path[])  [unwired: 6 in, 4 out]
        n150 = property class="Project"(reference=w318) -> ("Name"=w317:string)  [unwired: 1 in, 2 out]
        n151 = for {
          tunnel: w307 -> [w338] mode=indexing
          tunnel: [w337] -> w310 mode=indexing
          n152 = call <vilib>:"Get File Extension.vi"("file"=w338) -> ("filename without extension"=w337:string)  [unwired: 7 in, 3 out]
        }
        n153 = invoke class="VI" method="FP.Center"(reference=w306) -> ()  [unwired: 2 in, 3 out]
        n154 = Match Pattern(string=w317, regular expression=".lvproj") -> (before substring=w309:string)  [unwired: 1 in, 3 out]
        n155 = Search 1D Array(1D array=w310, element=w309) -> (index of element=w308:i32)  [unwired: 1 in]
        n156 = property class="MCListbox (strict)"(reference=w325, "ItemNames"=string[][] [] ("Item Names"), "Caption.Text"="Build Steps (0)", "SelColor"=u32 16777224) -> ()  [unwired: 1 in, 2 out]
        n157 = case shown="Default" w308 {
          selector: w308 -> [w330 _]
          tunnel: [w327 w333] -> w315
          tunnel: w309 -> [_ w332]
          tunnel: w307 -> [w331 _]
          tunnel: ["UI: Load" ("State(s) at Back (\"\")") _] -> w302
          frame Default {
            n158 = Index Array(array=w331, index=w330) -> (element=w329:path)
            n159 = Read from Binary File(5:refnum<class "CI Project.lvclass"> refnum ("CI Project out"), 11:w329) -> (2:w327:refnum<class "CI Project.lvclass">)  [unwired: 4 in, 3 out]
          }
          frame -1 {
            # "Used to capture default values from controls"
            n160 = local read "Jenkins Hostname(IP Address:Port Number)"() -> (w336:string)
            n161 = local read "Notification (Separate by Space)"() -> (w335:string)
            n162 = local read "How many days to Artifact?"() -> (w334:i32)
            n163 = local write "Project Name"(w332) -> ()
            n164 = call "Create.vi"("HostName"=w336, "Artifact Days"=w334, "Notification"=w335, "Project Name"=w332) -> ("CI Project out"=w333:refnum<class "CI Project.lvclass">)  [unwired: 6 in, 1 out]
          }
        }
        n165 = property class="Bool"(reference=w321, "DisabledEnum"=T5."Enabled" ("Disabled")) -> ()  [unwired: 1 in, 2 out]
        n166 = Bundle By Name(cluster=w314, "CI Project"=w315) -> (w313:T11)
        n167 = call-poly "QSM - Add State(s).vi"("QSM"=w305, "error in (no error)"=w304, "State(s)"=w302) -> ("error out"=w303:errorcluster)  [unwired: 8 in]
      }
      frame "UI: Add Build Step" {
        # "When Add:\n1. Add the Type to the List\n2. Add to data table\n3. Set the Label of Build Steps"
        n168 = Unbundle By Name(w352) -> ("Build Steps Data"=w350:variant, "Build Steps Ref"=w361:refnum<vi>, "Number of Build Steps"=w343:i32, "Step Type"=w342:enum16{"LabVIEW Build", "Run VI"})
        n169 = Format Into String(w342) -> (resulting string=w340:string)  [unwired: 3 in, 1 out]
        n170 = case shown="\"Run VI\"" w342 {
          tunnel: [enum32{"LabVIEW Build", "Run VI", "Blank"}."LabVIEW Build" ("Build Type Tab") enum32{"LabVIEW Build", "Run VI", "Blank"}."Run VI" ("Build Type Tab")] -> w341
          tunnel: [w367 w372] -> w339
          tunnel: w340 -> [w366 w373]
          frame "LabVIEW Build", Default {
            n171 = Set Variant Attribute(Variant=variant ("variant"), name=w366, value=T7 {"Executor_Number"="", "Workspace_Path"="", "Build_Spec"="", "Project_Path"="", "Auto_Version_Increment"=FALSE} ("LabVIEW Build")) -> (Variant out=w367:variant)  [unwired: 1 in, 2 out]
          }
          frame "Run VI" {
            n172 = Set Variant Attribute(Variant=variant ("variant"), name=w373, value=T8 {"Executor_Number"="", "VI_Path"="", "Wait_Until_Done"=FALSE} ("Run VI")) -> (Variant out=w372:variant)  [unwired: 1 in, 2 out]
          }
        }
        n173 = call "Get GUID.vi"() -> ("GUID"=w345:string)  [unwired: 11 in]
        n174 = Increment(x=w343) -> (x+1=w363:i32)
        n175 = property class="MCListbox (strict)"(reference=w361) -> (reference out=w354:refnum<vi>, "ItemNames"=w360:string[][])  [unwired: 1 in, 1 out]
        n176 = Format Into String(format string="%s:%s", w340, w345) -> (resulting string=w344:string)  [unwired: 2 in, 1 out]
        n177 = Concatenate Strings(w340, "()" ("string")) -> (w348:string)
        n178 = Format Into String(format string="Build Steps(%d)", w363) -> (resulting string=w362:string)  [unwired: 2 in, 1 out]
        n179 = Build Array(w348, w344) -> (w359:string[])
        n180 = for {
          N: w343 -> [_]
          shift-right: [w379] -> w353
          shift-left: w354 -> [w380]
          i -> [w376]
          n181 = Bundle By Name(cluster=T6 {"Row"=0, "Column"=0} ("Active Cell:Active Cell"), "Row"=w376) -> (w377:T6)
          n182 = property class="MCListbox (strict)"(reference=w380, "ActiveCell"=w377, "CellBG"=u32 16777225) -> (reference out=w379:refnum<vi>)  [unwired: 1 in, 1 out]
        }
        n183 = Build Array (concatenate)(w360, w359) -> (w358:string[][])
        n184 = Bundle By Name(cluster=T6 {"Row"=0, "Column"=0} ("Active Cell:Active Cell"), "Row"=w343) -> (w355:T6)
        n185 = Set Variant Attribute(Variant=w350, name=w344, value=w339) -> (Variant out=w349:variant)  [unwired: 1 in, 2 out]
        n186 = property class="MCListbox (strict)"(reference=w353, "ItemNames"=w358, "Caption.Text"=w362, "ActiveCell"=w355, "CellBG"=u32 16777224) -> ()  [unwired: 1 in, 2 out]
        n187 = Bundle By Name(cluster=w352, "Build Steps Data"=w349, "Active GUID"=w344, "Active Step Data"=w339, "Number of Build Steps"=w363, "Build Type Tab"=w341, "Build Step Index"=w343) -> (w351:T11)
      }
      frame "UI: Remove Build Step" {
        # "When Add:\n1. Add the Type to the List\n2. Add to data table\n3. Set the Label of Build Steps"
        n188 = Unbundle By Name(w396) -> ("Build Steps Data"=w394:variant, "Build Steps Ref"=w399:refnum<vi>, "Number of Build Steps"=w392:i32, "Build Step Index"=w388:i32)
        n189 = property class="MCListbox (strict)"(reference=w399) -> (reference out=w398:refnum<vi>, "ItemNames"=w391:string[][])  [unwired: 1 in, 1 out]
        n190 = Decrement(x=w392) -> (x-1=w401:i32)
        n191 = Format Into String(format string="Build Steps(%d)", w401) -> (resulting string=w400:string)  [unwired: 2 in, 1 out]
        n192 = Delete From Array(array=w391, length=1, index (row)=w388) -> (deleted portion=w387:string[][], array with subset deleted=w390:string[][])  [unwired: 1 in]
        n193 = for {
          N: w392 -> [_]
          shift-right: [w407] -> w397
          shift-left: w398 -> [w408]
          i -> [w404]
          n194 = Bundle By Name(cluster=T6 {"Row"=0, "Column"=0} ("Active Cell:Active Cell"), "Row"=w404) -> (w405:T6)
          n195 = property class="MCListbox (strict)"(reference=w408, "ActiveCell"=w405, "CellBG"=u32 16777225) -> (reference out=w407:refnum<vi>)  [unwired: 1 in, 1 out]
        }
        n196 = Index Array(array=w387, index (row)=0 ("disabled index (row)"), index (col)=1 ("disabled index (col)")) -> (element=w383:string)
        n197 = Delete Variant Attribute(6:w383, 7:w394) -> (3:w393:variant)  [unwired: 1 in, 2 out]
        n198 = property class="MCListbox (strict)"(reference=w397, "ItemNames"=w390, "Caption.Text"=w400) -> ()  [unwired: 1 in, 2 out]
        n199 = Bundle By Name(cluster=w396, "Build Steps Data"=w393, "Active Step Data"=variant ("variant"), "Number of Build Steps"=w401, "Build Type Tab"=enum32{"LabVIEW Build", "Run VI", "Blank"}."Blank", "Build Step Index"=w392) -> (w395:T11)
      }
      frame "UI: Update Indicators" {
        n200 = Unbundle By Name(w417) -> ("Main Tab"=w411:enum32{"Information", "Result Text"}, "Active Step Data"=w416:variant)
        n201 = Get Variant Attribute(Variant=w416) -> (names=w415:string[], values=w413:variant[])  [unwired: 3 in, 2 out]
        n202 = Index Array(array=w415) -> (element=w414:string)  [unwired: 1 in]
        n203 = Index Array(array=w413) -> (element=w412:variant)  [unwired: 1 in]
        n204 = case shown="\"Run VI\"" w414 {
          tunnel: [enum32{"LabVIEW Build", "Run VI", "Blank"}."Blank" ("Build Type Tab") enum32{"LabVIEW Build", "Run VI", "Blank"}."LabVIEW Build" ("Build Type Tab") enum32{"LabVIEW Build", "Run VI", "Blank"}."Run VI" ("Build Type Tab")] -> w410
          tunnel: w412 -> [_ w434 w442]
          frame Default {
          }
          frame "LabVIEW Build" {
            n205 = property class="App"() -> ("Project"=w427:refnum<vi>[])  [unwired: 2 in, 2 out]
            n206 = Variant To Data(type=T7 {"Executor_Number"="", "Workspace_Path"="", "Build_Spec"="", "Project_Path"="", "Auto_Version_Increment"=FALSE} ("LabVIEW Build"), Variant=w434) -> (data=w432:T7)  [unwired: 1 in, 1 out]
            n207 = Unbundle By Name(w432) -> ("Project_Path"=w429:string, "Build_Spec"=w431:string)
            n208 = Index Array(array=w427) -> (element=w426:refnum<vi>)  [unwired: 1 in]
            n209 = property class="Project"(reference=w426) -> ("Path"=w424:path)  [unwired: 1 in, 2 out]
            n210 = String To Path(string=w429) -> (path=w423:path)
            n211 = Empty String/Path?(string/path=w423) -> (empty?=w425:bool)
            n212 = Select(t=w424, s=w425, f=w423) -> (s? t:f=w421:path)
            n213 = call <vilib>:"GetTargetBuildSpecs.vi"("Path to project"=w421) -> ("buildspec refs"=w430:refnum<vi>[])  [unwired: 8 in, 2 out]
            n214 = for {
              tunnel: w430 -> [w436] mode=indexing
              tunnel: [w435] -> w428 mode=indexing
              n215 = property class="ProjectItem"(reference=w436) -> ("Name"=w435:string)  [unwired: 1 in, 2 out]
            }
            n216 = property on="Build Spec" class="Ring (strict)"("Strings []"=w428) -> ()  [unwired: 2 in, 2 out]
            n217 = local write "Project Path"(w421) -> ()
            n218 = Search 1D Array(1D array=w428, element=w431) -> (index of element=w420:i32)  [unwired: 1 in]
            n219 = local write "Build Spec"(w420) -> ()
          }
          frame "Run VI" {
            n220 = Variant To Data(type=T8 {"Executor_Number"="", "VI_Path"="", "Wait_Until_Done"=FALSE} ("Run VI"), Variant=w442) -> (data=w440:T8)  [unwired: 1 in, 1 out]
            n221 = Unbundle By Name(w440) -> ("VI_Path"=w439:string, "Wait_Until_Done"=w437:bool)
            n222 = String To Path(string=w439) -> (path=w438:path)
            n223 = local write "VI Path"(w438) -> ()
            n224 = local write "Wait Until Done?"(w437) -> ()
          }
        }
        "Build Type Tab" <- w410
        n225 = local write "Main Tab"(w411) -> ()
      }
      frame "UI: Update List Name" {
        w457 = 0 ("disabled index (col)")
        n226 = Unbundle By Name(w445) -> ("Build Steps Ref"=w459:refnum<vi>, "Build Step Index"=w456:i32, "List Text"=w446:string)
        n227 = property class="MCListbox (strict)"(reference=w459) -> (reference out=w449:refnum<vi>, "ItemNames"=w458:string[][])  [unwired: 1 in, 1 out]
        n228 = Index Array(array=w458, index (row)=w456, index (col)=w457) -> (element=w452:string)
        n229 = Match Pattern(string=w452, regular expression="(") -> (offset past match=w444:i32)  [unwired: 1 in, 3 out]
        n230 = Match Pattern(string=w452, regular expression=")") -> (offset past match=w453:i32)  [unwired: 1 in, 3 out]
        n231 = Subtract(x=w453, y=w444) -> (x-y=w448:i32)
        n232 = Decrement(x=w448) -> (x-1=w447:i32)
        n233 = Replace Substring(2:w447, 3:w444, 4:w446, 5:w452) -> (1:w451:string)  [unwired: 1 out]
        n234 = Replace Array Subset(array=w458, new element=w451, index (row)=w456, index (col)=w457) -> (w450:string[][])
        n235 = property class="MCListbox (strict)"(reference=w449, "ItemNames"=w450) -> ()  [unwired: 1 in, 2 out]
      }
      frame "UI: Load" {
        n236 = Unbundle By Name(w485) -> ("Build Steps Ref"=w477:refnum<vi>, "Build Steps Data"=w479:variant, "CI Project"=w486:refnum<class "CI Project.lvclass">)
        n237 = property class="CI Project.lvclass"(reference=w486) -> ("Build Recipe"=w473:refnum<class "Build Job.lvclass">[], "Project Name"=w471:string, "Artifact Days"=w470:i32, "HostName"=w469:string, "Notification"=w468:string)  [unwired: 1 in, 2 out]
        n238 = local write "Jenkins Hostname(IP Address:Port Number)"(w469) -> ()
        n239 = local write "Project Name"(w471) -> ()
        n240 = local write "How many days to Artifact?"(w470) -> ()
        n241 = local write "Notification (Separate by Space)"(w468) -> ()
        n242 = Delete From Array(array=w473, length=1, index=0) -> (deleted portion=w467:refnum<class "Build Job.lvclass">[], array with subset deleted=w472:refnum<class "Build Job.lvclass">[])
        n243 = for {
          tunnel: w472 -> [w498] mode=indexing
          tunnel: [w497] -> w482
          shift-right: [w494] -> w478
          shift-left: w479 -> [w496]
          tunnel: [w488] -> w476 mode=indexing
          i -> [w497]
          n244 = call "Get GUID.vi"() -> ("GUID"=w499:string)  [unwired: 11 in]
          n245 = call "Get Class Name.vi"("lvclass"=w498) -> ("Class Name"=w492:string)  [unwired: 10 in]
          n246 = call-dynamic "Class to Variant.vi"("Build Job in"=w498) -> ("Display"=w491:string, "Data"=w495:variant)  [unwired: 7 in, 2 out]
          n247 = Format Into String(format string="%s:%s", w492, w499) -> (resulting string=w489:string)  [unwired: 2 in, 1 out]
          n248 = Set Variant Attribute(Variant=w496, name=w489, value=w495) -> (Variant out=w494:variant)  [unwired: 1 in, 2 out]
          n249 = Format Into String(format string="%s(%s)", w492, w491) -> (resulting string=w490:string)  [unwired: 2 in, 1 out]
          n250 = Build Array(w490, w489) -> (w488:string[])
        }
        n251 = Index Array(array=w467) -> (element=w466:refnum<class "Build Job.lvclass">)  [unwired: 1 in]
        n252 = To More Specific Class(target class=refnum<class "Job Initialize.lvclass"> refnum ("Job Initialize out"), reference=w466) -> (specific class reference=w464:refnum<class "Job Initialize.lvclass">)  [unwired: 1 in, 1 out]
        n253 = property class="Job Initialize.lvclass"(reference=w464) -> ("Build Trigger"=w463:T2, "Source Code Poll"=w462:T1)  [unwired: 1 in, 2 out]
        n254 = Increment(x=w482) -> (x+1=w480:i32)
        n255 = Format Into String(format string="Build Steps(%d)", w480) -> (resulting string=w475:string)  [unwired: 2 in, 1 out]
        n256 = property class="MCListbox (strict)"(reference=w477, "ItemNames"=w476, "Caption.Text"=w475) -> ()  [unwired: 1 in, 2 out]
        n257 = local write "Build Trigger"(w463) -> ()
        n258 = local write "Source Code Poll"(w462) -> ()
        n259 = Bundle By Name(cluster=w485, "Build Steps Data"=w478, "Active Step Data"=variant, "Number of Build Steps"=w480) -> (w484:T11)
      }
      frame "---------- Macro ----------" {
        # "Do not put any code in this frame.\n(It is a separator no-op. You can make a copy of this frame to create a new Macro frame)"
      }
      frame "Macro: Initialize" {
        # "Initialization Macro\n(This is called once, when the VI starts)"
        n260 = call-poly "QSM - Add State(s).vi"("QSM"=w506, "error in (no error)"=w505, "State(s)"="Data: Initialize\nInitialize Core Data\nUI: Main Info\nUI: Initialize\nUI: Update Indicators") -> ("error out"=w504:errorcluster)  [unwired: 8 in]
      }
      frame "Macro: Build" {
        n261 = call-poly "QSM - Add State(s).vi"("QSM"=w511, "error in (no error)"=w510, "State(s)"="Build: Initialize\nBuild: Assemble\nSave\nBuild: Send" ("State(s) at Back (\"\")")) -> ("error out"=w509:errorcluster)  [unwired: 8 in]
      }
      frame "Macro: Exit" {
        # "Exit Macro\n(This is called once, when the VI exits)"
        n262 = call-poly "QSM - Add State(s).vi"("QSM"=w516, "error in (no error)"=w515, "State(s)"="Data: Cleanup\nExit") -> ("error out"=w514:errorcluster)  [unwired: 8 in]
      }
      frame "---------- Build CI Project ----------" {
        # "Template Separator\n(You can make a copy of, or modify, this frame)"
      }
      frame "Build: Initialize" {
        n263 = Unbundle By Name(w522) -> ("CI Project"=w521:refnum<class "CI Project.lvclass">)
        n264 = Unbundle By Name(w528) -> ("Build Done? Event"=w527:refnum<user-event>)
        n265 = call "Build Events.vi"("error in (no error)"=w526, "CI Project in"=w521) -> ("error out"=w525:errorcluster, "Build Events"=w524:refnum<user-event>, "CI Project out"=w523:refnum<class "CI Project.lvclass">)  [unwired: 7 in]
        n266 = call <vilib>:"Set Busy.vi"("error in (no error)"=w525, "disable click? (T)"=FALSE) -> ("error out"=w529:errorcluster)  [unwired: 8 in, 1 out]
        n267 = register-events(w524, w527) -> (reference out=w520:refnum<event-registration>)  [unwired: 2 in, 1 out]
        n268 = Bundle By Name(cluster=w522, "CI Project"=w523, "Build Events"=w520) -> (w531:T11)
      }
      frame "Build: Assemble" {
        # "Account for Folder\nCreation"
        # "Your code here.\n(You can make a copy of, or modify, this frame)"
        n269 = Unbundle By Name(w537) -> ("CI Project"=w545:refnum<class "CI Project.lvclass">, "Build Steps Data"=w542:variant, "Build Steps Ref"=w544:refnum<vi>)
        n270 = property class="MCListbox (strict)"(reference=w544) -> ("ItemNames"=w543:string[][])  [unwired: 1 in, 2 out]
        n271 = for {
          tunnel: w543 -> [w558] mode=indexing
          tunnel: w542 -> [w556]
          tunnel: [w549] -> w535 mode=indexing if=w548
          n272 = Index Array(array=w558, index=1) -> (element=w555:string)
          n273 = Get Variant Attribute(Variant=w556, name=w555) -> (value=w554:variant)  [unwired: 2 in, 3 out]
          n274 = Get Variant Attribute(Variant=w554) -> (names=w553:string[], values=w552:variant[])  [unwired: 3 in, 2 out]
          n275 = Index Array(array=w552) -> (element=w550:variant)  [unwired: 1 in]
          n276 = Index Array(array=w553) -> (element=w551:string)  [unwired: 1 in]
          n277 = case shown="\"Run VI\"" w551 {
            tunnel: w550 -> [_ w565 w573]
            tunnel: [refnum<class "Build Job.lvclass"> refnum ("Build Job.lvclass") w564 w571] -> w549
            tunnel: [_ w560 w567] -> w548
            frame Default {
            }
            frame "LabVIEW Build" {
              n278 = Variant To Data(type=T7 {"Executor_Number"="", "Workspace_Path"="", "Build_Spec"="", "Project_Path"="", "Auto_Version_Increment"=FALSE} ("LabVIEW Build"), Variant=w565) -> (data=w563:T7)  [unwired: 1 in, 1 out]
              n279 = Unbundle By Name(w563) -> ("Build_Spec"=w562:string)
              n280 = call "Create.vi"("LabVIEW Build"=w563) -> ("LabVIEW Build out"=w564:refnum<class "LabVIEW Build.lvclass">)  [unwired: 9 in, 1 out]
              n281 = Empty String/Path?(string/path=w562) -> (empty?=w561:bool)
              n282 = Not(x=w561) -> (.not. x?=w560:bool)
            }
            frame "Run VI" {
              n283 = Variant To Data(type=T8 {"Executor_Number"="", "VI_Path"="", "Wait_Until_Done"=FALSE} ("Run VI"), Variant=w573) -> (data=w570:T8)  [unwired: 1 in, 1 out]
              n284 = Unbundle By Name(w570) -> ("VI_Path"=w569:string)
              n285 = call "Create.vi"("Run VI"=w570) -> ("Run VI out"=w571:refnum<class "Run VI.lvclass">)  [unwired: 9 in, 1 out]
              n286 = Empty String/Path?(string/path=w569) -> (empty?=w568:bool)
              n287 = Not(x=w568) -> (.not. x?=w567:bool)
            }
          }
        }
        n288 = call "Create.vi"("Source Code Poll"="Source Code Poll", "Build Trigger"="Build Trigger") -> ("Job Initialize out"=w541:refnum<class "Job Initialize.lvclass">)  [unwired: 8 in, 1 out]
        n289 = Build Array (concatenate)(w541, w535) -> (w534:refnum<class "Build Job.lvclass">[])
        n290 = Array Size(array=w534) -> (size(s)=w532:i32)
        n291 = To Double Precision Float(number=w532) -> (double precision float=w533:dbl)
        n292 = call "Add Build Recipe.vi"("error in (no error)"=w540, "Build Recipe"=w534, "CI Project in"=w545) -> ("error out"=w539:errorcluster, "CI Project out"=w538:refnum<class "CI Project.lvclass">)  [unwired: 7 in]
        n293 = property on="Progress" class="Slide (strict)"("Scale.Maximum"=w533) -> ()  [unwired: 2 in, 2 out]
        n294 = Bundle By Name(cluster=w537, "CI Project"=w538, "Jenkins Steps"=w532) -> (w536:T11)
      }
      frame "Build: Send" {
        n295 = Unbundle By Name(w575) -> ("Jenkins Builder Enquerer"=w574:refnum<class "Message Enqueuer.lvclass">)
        n296 = Unbundle By Name(w579) -> ("CI Project"=w578:refnum<class "CI Project.lvclass">)
        n297 = call "Send Build.vi"("error in (no error)"=w577, "CI Project"=w578, "Message Enqueuer"=w574) -> ("error out"=w576:errorcluster)  [unwired: 7 in, 1 out]
      }
      frame "Save" {
        n298 = Unbundle By Name(w592) -> ("CI Project"=w591:refnum<class "CI Project.lvclass">)
        n299 = Unbundle By Name(w593) -> ("Projects Path"=w590:path)
        n300 = property class="CI Project.lvclass"(reference=w591) -> (reference out=w586:refnum<class "CI Project.lvclass">, "Project Name"=w588:string)  [unwired: 1 in, 1 out]
        n301 = Format Into String(format string="%s.jenk", w588) -> (resulting string=w587:string)  [unwired: 2 in, 1 out]
        n302 = Build Path(base path=w590, name or relative path=w587) -> (appended path=w585:path)
        n303 = Open/Create/Replace File(file path (use dialog)=w585, error in=w582, operation (0:open)=T10."replace or create") -> (refnum out=w584:refnum<file>, error out=w581:errorcluster)  [unwired: 3 in, 1 out]
        n304 = Write to Binary File(file (use dialog)=w584, data=w586, error in=w581) -> (error out=w580:errorcluster)  [unwired: 3 in, 2 out]
        n305 = case shown="No Error" w580 {
          frame No Error {
            n306 = One Button Dialog(message="Project Saved Successfully") -> ()  [unwired: 1 in, 1 out]
          }
          frame Error {
          }
        }
      }
    }
  }
